vi "Progress bar.vi"(11 "Numeric":i32) -> (3 "Boolean Array":bool[](array[boolean]))   [LabVIEW 2014]
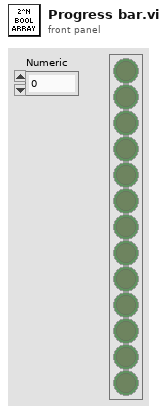
[diagram p1: front panel]
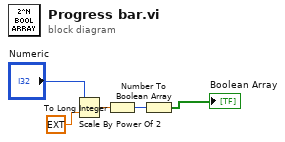
[diagram p0: block diagram]
diagram:
  n1 = Scale By Power Of 2(n="Numeric", x=ext 1.0) -> (x*2^n=w3:ext)
  n2 = To Long Integer(number=w3) -> (32bit integer=w4:i32)
  n3 = Number To Boolean Array(number=w4) -> (Boolean array=→"Boolean Array":bool[])
